vi "Unflatten FIFO Config.vi"(8 "error in":errorcluster, 10 "Flattened Data in":u8[](array[numeric]), 11 "FIFO Config in":T1) -> (0 "error out":errorcluster, 2 "Flatten Data out":u8[](array[numeric]), 3 "FIFO Config out":T1)   [LabVIEW 2021, in "ChannelCommon.lvlib"]
uses:
  ChannelCommon.lvlib
  typedef/FIFO Config.ctl
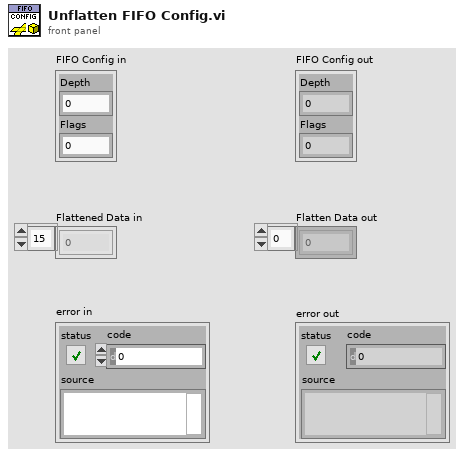
[diagram p1: front panel]
types:
  T1 = typedef "ChannelCommon.lvlib/FIFO Config.ctl" = cluster{"Depth":u64, "Flags":u64}
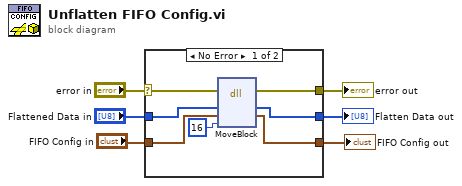
[diagram p0: block diagram]
diagram:
  n1 = case shown="No Error" "error in" {
    selector: "error in" -> [w7 w16]
    tunnel: "FIFO Config in" -> [w13 w14]
    tunnel: "Flattened Data in" -> [w12 w15]
    tunnel: [w11 w16] -> w5
    tunnel: [w10 w14] -> w1
    tunnel: [w9 w15] -> w4
    frame No Error {
      n2 = dll-call lib="LabVIEW" fn="MoveBlock"(error in=w7, "source"=w12, "dest"=w13, "size"=u64 16) -> (error out=w11:errorcluster, "source"=w9:u8[], "dest"=w10:T1)  [unwired: 4 in, 1 out]
    }
    frame Error {
    }
  }
  "error out" <- w5
  "Flatten Data out" <- w4
  "FIFO Config out" <- w1
